vi "ConverteTipoSinalParaString.vi"(2 "Tipo":T1) -> (16 "String":string)   [LabVIEW 2017]
uses:
  Typedefs/Tipo_TipoSinalSimulado.ctl
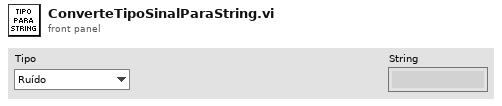
[diagram p1: front panel]
types:
  T1 = typedef "Tipo_TipoSinalSimulado.ctl" = enum16{"Ruído", "Fasor", "Senóide", "Composto", "AM", "Proximidade", "Entreferro"}
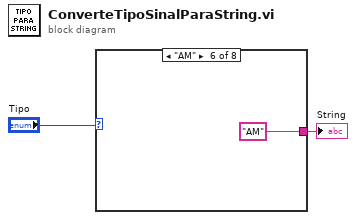
[diagram p0: block diagram]
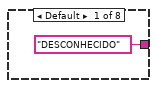
[diagram p2: hidden frame]
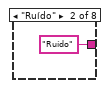
[diagram p3: hidden frame]
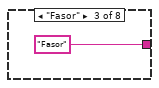
[diagram p4: hidden frame]
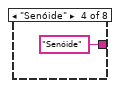
[diagram p5: hidden frame]
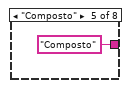
[diagram p6: hidden frame]
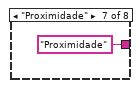
[diagram p7: hidden frame]
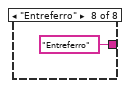
[diagram p8: hidden frame]
diagram:
  n1 = case shown="\"AM\"" "Tipo" {
    tunnel: ["DESCONHECIDO" "Ruído" "Fasor" "Senóide" "Composto" "AM" "Proximidade" "Entreferro"] -> w1
    frame Default {
    }
    frame "Ruído" {
    }
    frame "Fasor" {
    }
    frame "Senóide" {
    }
    frame "Composto" {
    }
    frame "AM" {
    }
    frame "Proximidade" {
    }
    frame "Entreferro" {
    }
  }
  "String" <- w1
